vi "Connect Interface Sessions.vi"(8 "error in (no error)":errorcluster, 11 "PXImc Transceiver in":refnum<class "PXImc Transceiver.lvclass">) -> (0 "error out":errorcluster, 3 "PXImc Transceiver out":refnum<class "PXImc Transceiver.lvclass">)   [LabVIEW 2017, in "PXImc.lvlib" / "PXImc Transceiver.lvclass"]
uses:
  PXImc Transceiver.lvclass
  <vilib>/pximc/Connect (U8).vi
  <vilib>/pximc/nipximc.lvlib
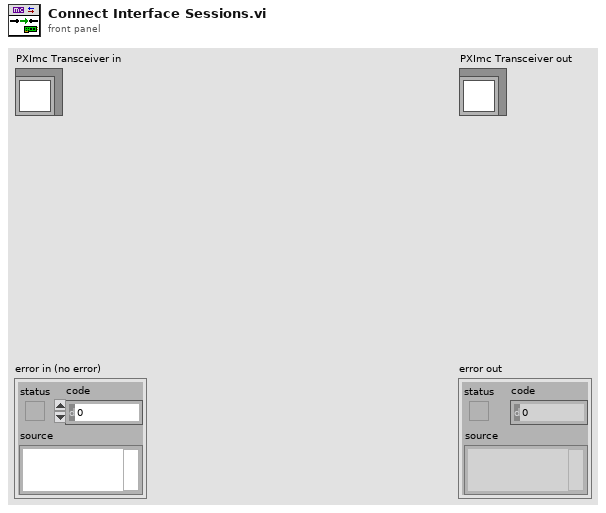
[diagram p1: front panel]
types:
  T1 = typedef "PXImc.lvlib/PXImc Transceiver.lvclass/PXImc Transfer Data.ctl" = cluster{"stream id":u16, "session":refnum<k21>, "buffer size":u64}
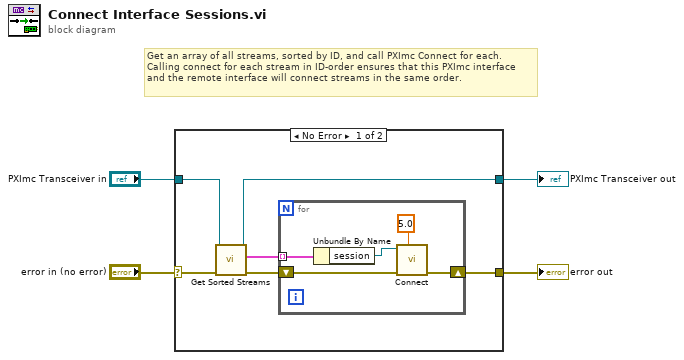
[diagram p0: block diagram]
diagram:
  # "Get an array of all streams, sorted by ID, and call PXImc Connect for each. Calling connect for each stream in ID-order ensures that this PXImc interface and the remote interface will connect streams in the same order."
  n1 = case shown="No Error" "error in (no error)" {
    selector: "error in (no error)" -> [w9 w17]
    tunnel: [w10 w17] -> w3
    tunnel: [w5 w16] -> w1
    tunnel: "PXImc Transceiver in" -> [w6 w16]
    frame No Error {
      n2 = call "Get Sorted Streams.vi"("error in (no error)"=w9, "PXImc Transceiver in"=w6) -> ("error out"=w8:errorcluster, "stream-sorted transfers"=w7:T1[], "PXImc Transceiver out"=w5:refnum<class "PXImc Transceiver.lvclass">)  [unwired: 7 in]
      n3 = for {
        shift-right: [w14] -> w10
        shift-left: w8 -> [w15]
        tunnel: w7 -> [w13] mode=indexing
        n4 = Unbundle By Name(w13) -> ("session"=w12:refnum<k21>)
        n5 = call-poly <vilib>:"Connect.vi"("timeout in seconds (-1)"=5.0, "error in (no error)"=w15, "session in"=w12) -> ("error out"=w14:errorcluster)  [unwired: 7 in, 1 out]
      }
    }
    frame Error {
    }
  }
  "error out" <- w3
  "PXImc Transceiver out" <- w1
